vi "RT Loop - Pumps.vi"(11 "Message Queue":refnum<queue>) -> ()   [LabVIEW 2018]
doc: "This Control Loop VI performs control calculations of diverter line (DL) rotation."
uses:
  Support/Message Queue/Message Cluster.ctl
  Support/Message Queue/Message.ctl
  <vilib>/Platform/TimedLoop/XDataNode/timing_clust.ctl
  <vilib>/Platform/TimedLoop/XDataNode/nitl_modes.ctl
  <vilib>/Platform/TimedLoop/XDataNode/wakeup.ctl
  Controls/Pumps State.ctl
  <vilib>/Platform/TimedLoop/XDataNode/loadnilvce.vi
  Globals/Global - RT Channels.vi
  <vilib>/Platform/TimedLoop/XDataNode/XDataNode.xnode
  <vilib>/Platform/TimedLoop/XDataNode/XDNodeRunTimeDep.lvlib
  support/Message Queue/Message Queue.lvlib
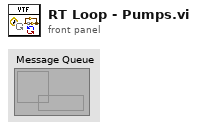
[diagram p1: front panel]
types:
  T1 = typedef "XDNodeRunTimeDep.lvlib/timing_clust.ctl" = cluster{"Expected End [f-1]":u64, "Actual End [f-1]":u64, "Finished Late? [f-1]":bool, "Expected End [i-1]":u64, "Actual End [i-1]":u64, "Finished Late? [i-1]":bool, "Expected Start [i]":u64, "Actual Start [i]":u64, "Expected Start [f]":u64, "Actual Start [f]":u64, "Source Name":string, "Structure Name":string, "Period":i64, "Deadline":i64, "Offset":i64, "Start":i64, "Priority":i32, "Timeout":i32, "Mode":T2, "Wakeup Reason":T3, "Error":errorcluster, "Source Type":string, "Secondary Source Type":string, "Global End Time":u64, "Global Start Time":u64, "Frame Duration":u64, "Iteration Duration":u64, "Assigned CPU":i32, "I/O Scan Engine Mode":u32}
  T2 = typedef "XDNodeRunTimeDep.lvlib/nitl_modes.ctl" = enum32{"No Change", "Process missed periods, maintain original phase", "Discard missed periods, maintain original phase", "Process missed periods, ignore original phase", "Discard missed periods, ignore original phase"}
  T3 = typedef "XDNodeRunTimeDep.lvlib/wakeup.ctl" = enum32{"Normal", "Aborted", "Asynchronous wakeup", "Timing source error", "Timed loop error", "Timeout"}
  T4 = typedef "Pumps State.ctl" = enum16{"Do Nothing", "Run Pump 1", "Run Pump 2", "Run Pump 3", "Run Pump 4", "Run Pump 5", "Stop Pump 1", "Stop Pump 2", "Stop Pump 3", "Stop Pump 4", "Stop Pump 5"}
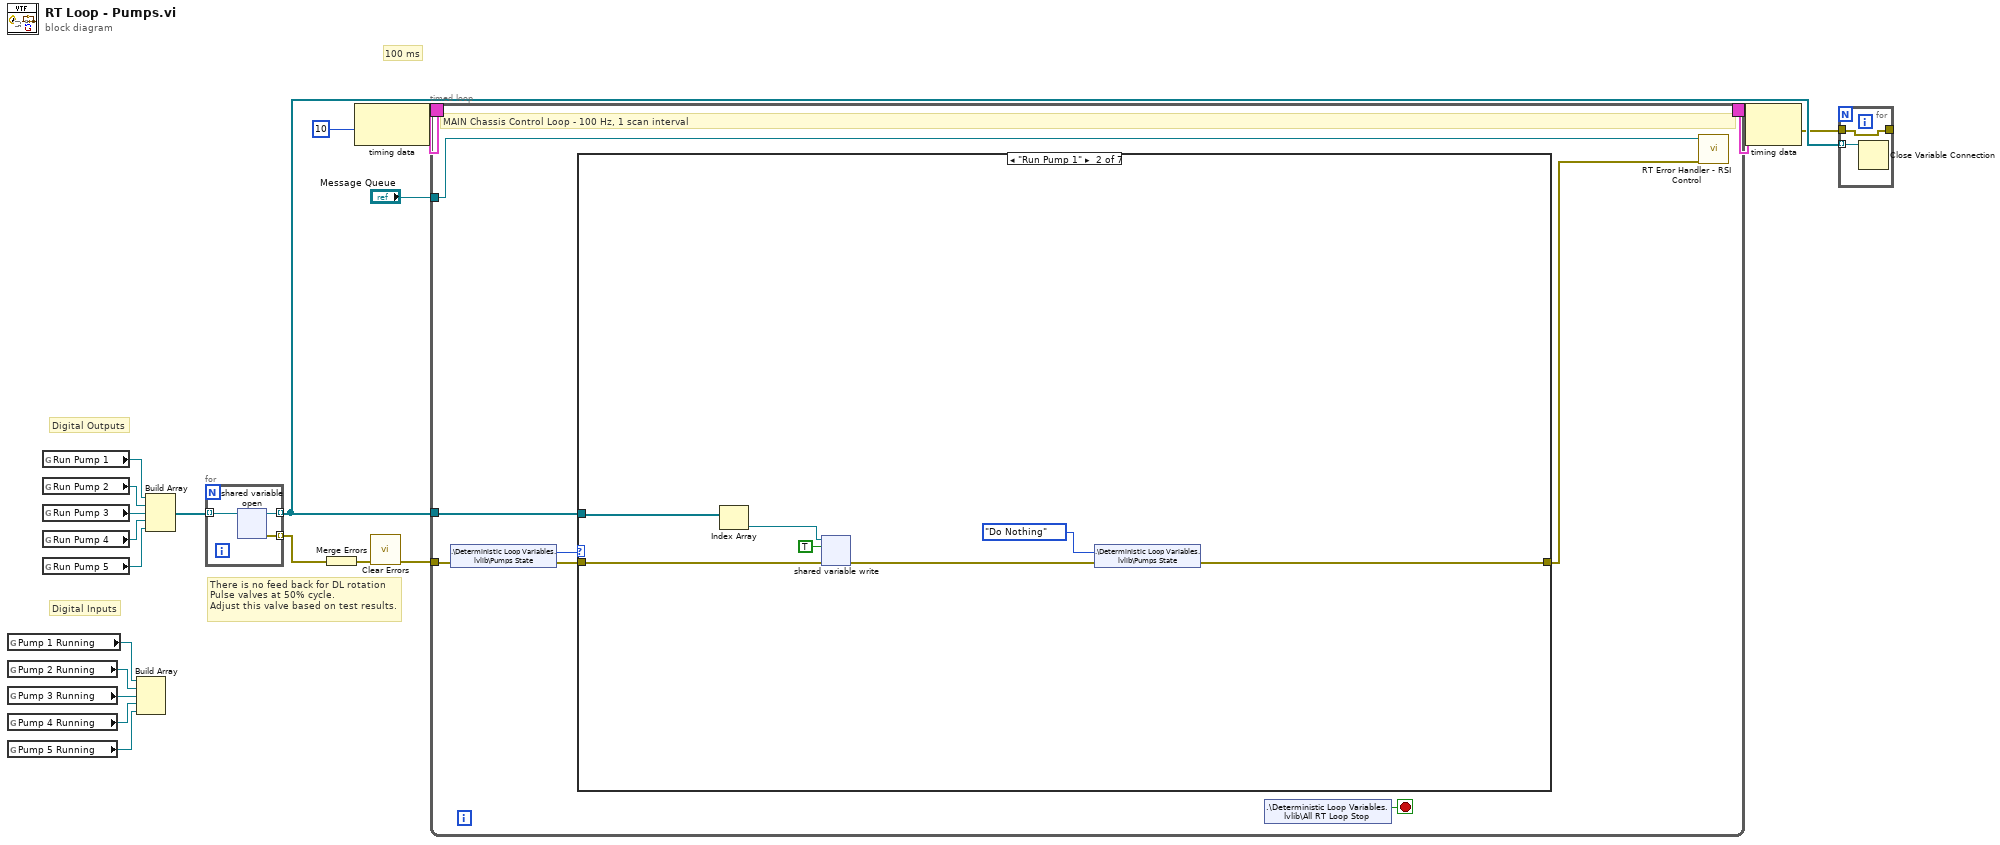
[diagram p0: block diagram]
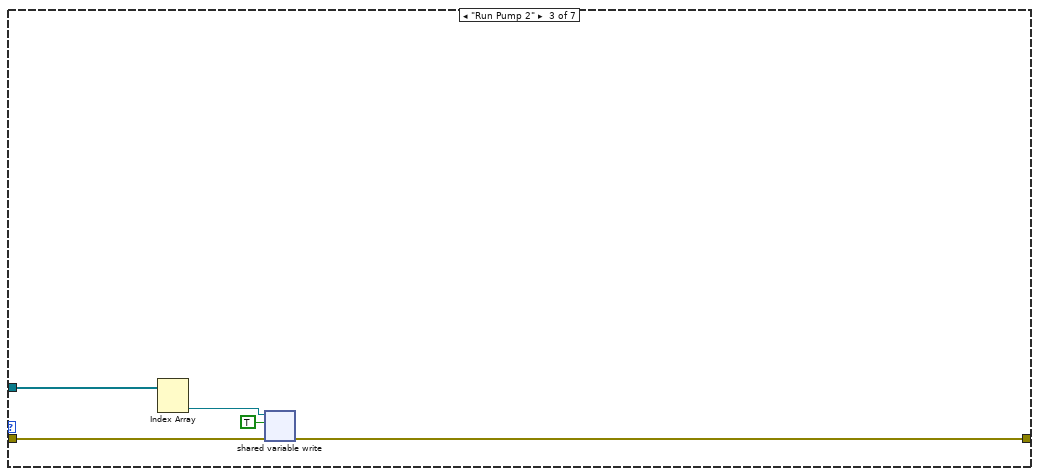
[diagram p3: hidden frame]
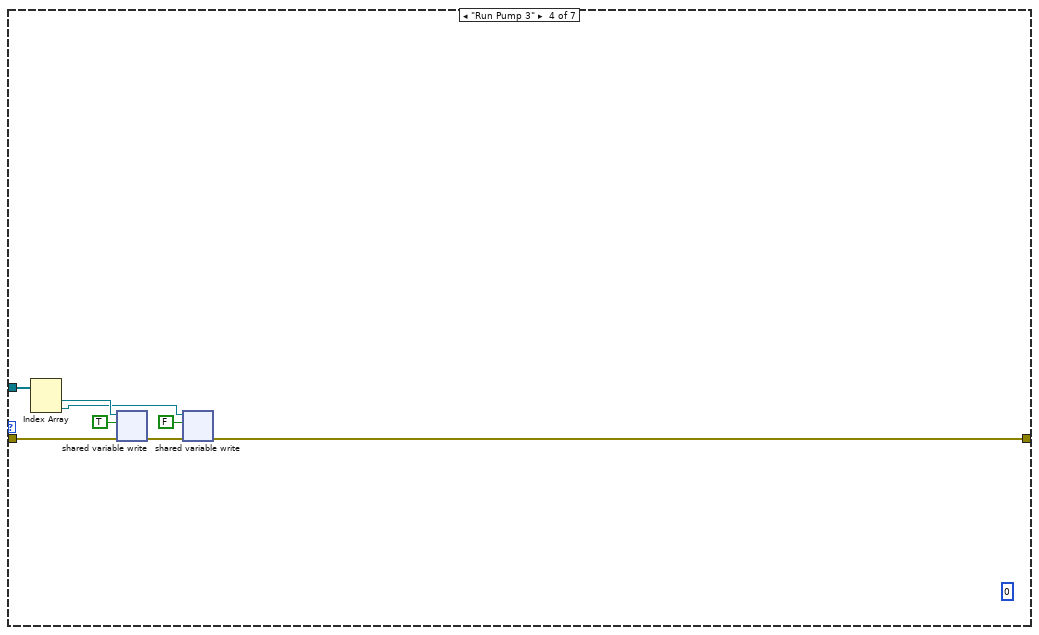
[diagram p4: hidden frame]
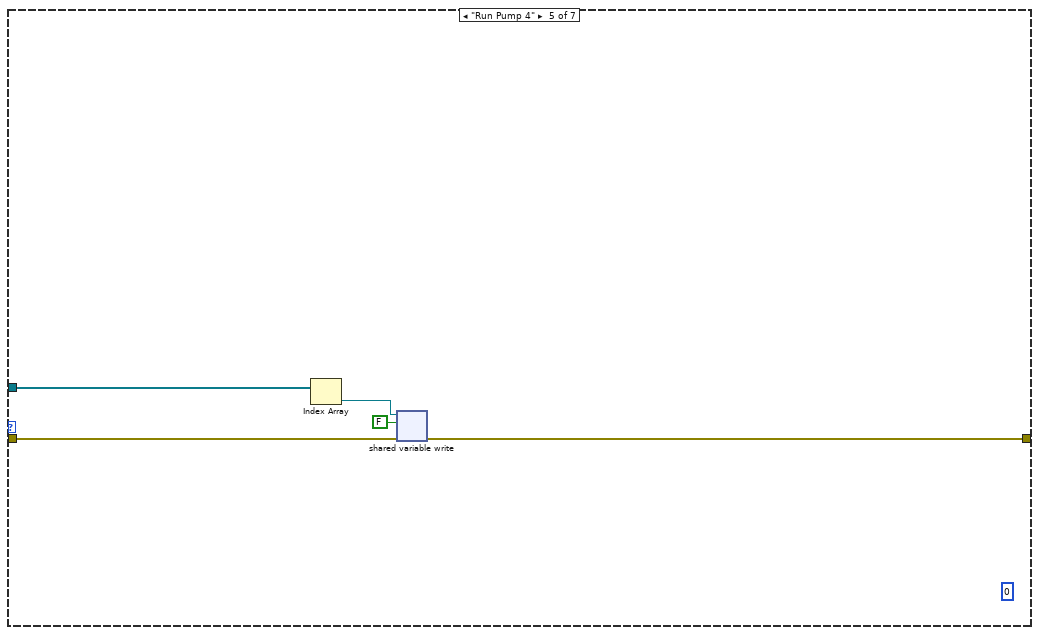
[diagram p5: hidden frame]
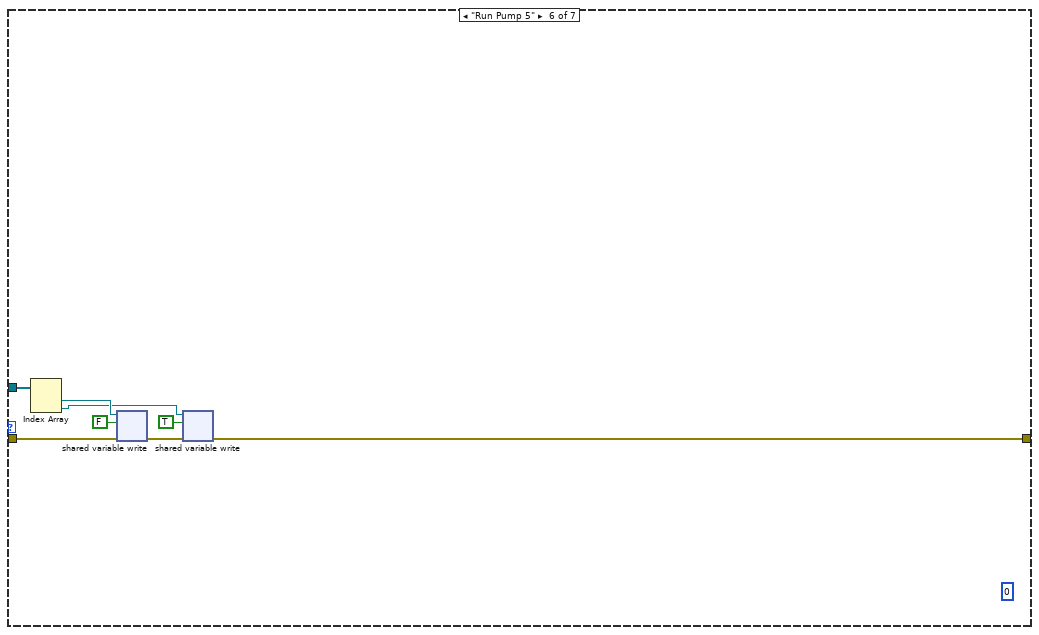
[diagram p6: hidden frame]
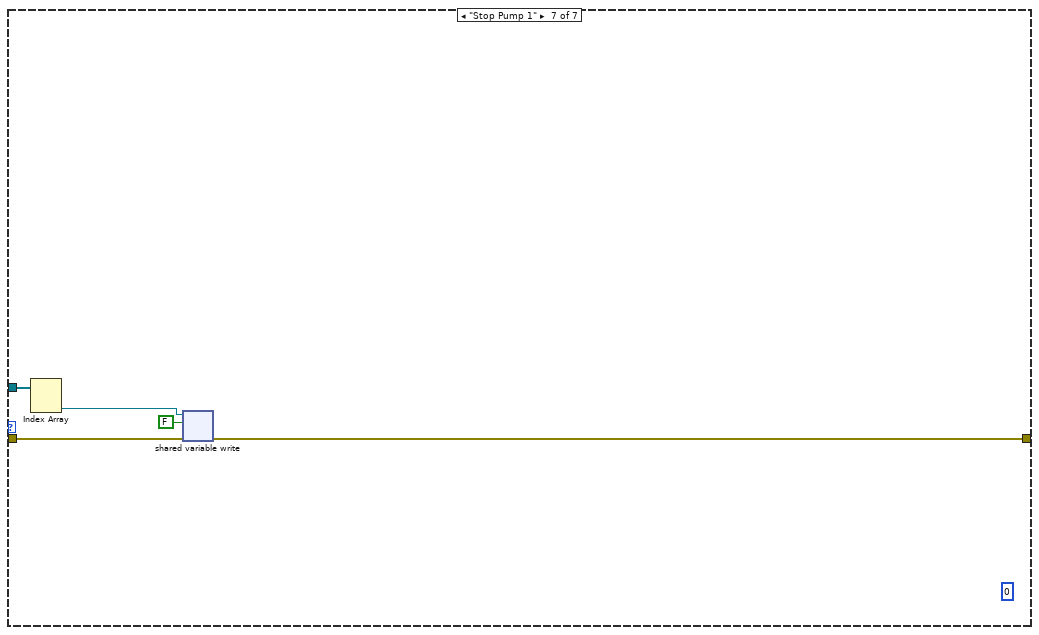
[diagram p7: hidden frame]
diagram:
  # "100 ms"
  # "Digital Inputs"
  # "There is no feed back for DL rotation\nPulse valves at 50% cycle. \nAdjust this valve based on test results."
  # "Digital Outputs"
  n1 = global read "Global - RT Channels.vi" "Pump 1 Running"() -> (w1:refnum<k21>)
  n2 = global read "Global - RT Channels.vi" "Pump 2 Running"() -> (w2:refnum<k21>)
  n3 = global read "Global - RT Channels.vi" "Pump 3 Running"() -> (w3:refnum<k21>)
  n4 = global read "Global - RT Channels.vi" "Pump 4 Running"() -> (w4:refnum<k21>)
  n5 = global read "Global - RT Channels.vi" "Pump 5 Running"() -> (w5:refnum<k21>)
  n6 = global read "Global - RT Channels.vi" "Run Pump 1"() -> (w11:refnum<k21>)
  n7 = global read "Global - RT Channels.vi" "Run Pump 2"() -> (w10:refnum<k21>)
  n8 = global read "Global - RT Channels.vi" "Run Pump 3"() -> (w9:refnum<k21>)
  n9 = global read "Global - RT Channels.vi" "Run Pump 4"() -> (w8:refnum<k21>)
  n10 = global read "Global - RT Channels.vi" "Run Pump 5"() -> (w7:refnum<k21>)
  n11 = Build Array(w1, w2, w3, w4, w5) -> ()  [unwired: 1 out]
  n12 = Build Array(w11, w10, w9, w8, w7) -> (w6:refnum<k21>[])
  n13 = for {
    tunnel: w6 -> [w23] mode=indexing
    tunnel: [w22] -> w15 mode=indexing
    tunnel: [w21] -> w12 mode=indexing
    n14 = shared-variable-open(w23) -> (w22:refnum<k21>, w21:errorcluster)  [unwired: 1 in]
  }
  n15 = Merge Errors(w12) -> (w13:errorcluster)
  n16 = node-c288(i64 10 ("Period")) -> (w20:T1)
  n17 = call <vilib>:"Clear Errors.vi"("error in (no error)"=w13) -> ("error out"=w16:errorcluster)  [unwired: 5 in, 1 out]
  n18 = timed-loop {
    timing: w20 -> [_]
    timing-out: [_] -> w19
    tunnel: "Message Queue" -> [w25]
    tunnel: w16 -> [w27]
    tunnel: w15 -> [w29]
    stop <- w30 stop-if-true
    # "MAIN Chassis Control Loop - 100 Hz, 1 scan interval"
    n19 = shared-variable ".\\Deterministic Loop Variables.lvlib\\Pumps State"(error in=w27) -> (w28:T4, error out=w26:errorcluster)
    n20 = case shown="\"Run Pump 1\"" w28 {
      tunnel: w29 -> [_ w38 w42 w51 w56 w64 w69]
      tunnel: w26 -> [w31 w36 w40 w48 w54 w61 w67]
      tunnel: [w31 w33 w43 w44 w53 w57 w66] -> w24
      frame "Do Nothing", Default {
      }
      frame "Run Pump 1" {
        n21 = Index Array(array=w38) -> (element=w37:refnum<k21>)  [unwired: 1 in]
        n22 = shared-variable-write(w37, w36, TRUE ("data in")) -> (w34:errorcluster)  [unwired: 1 out]
        n23 = shared-variable ".\\Deterministic Loop Variables.lvlib\\Pumps State"(Pumps_State."Do Nothing" ("Pumps State"), error in=w34) -> (error out=w33:errorcluster)
      }
      frame "Run Pump 2" {
        n24 = Index Array(array=w42) -> (element #2=w41:refnum<k21>)  [unwired: 2 in, 1 out]
        n25 = shared-variable-write(w41, w40, TRUE ("data in")) -> (w43:errorcluster)  [unwired: 1 out]
      }
      frame "Run Pump 3" {
        (unwired) 0
        n26 = Index Array(array=w51) -> (element #1=w50:refnum<k21>, element #2=w49:refnum<k21>)  [unwired: 2 in]
        n27 = shared-variable-write(w50, w48, TRUE ("data in")) -> (w47:errorcluster)  [unwired: 1 out]
        n28 = shared-variable-write(w49, w47, FALSE ("data in")) -> (w44:errorcluster)  [unwired: 1 out]
      }
      frame "Run Pump 4" {
        (unwired) 0
        n29 = Index Array(array=w56) -> (element=w55:refnum<k21>)  [unwired: 1 in]
        n30 = shared-variable-write(w55, w54, FALSE ("data in")) -> (w53:errorcluster)  [unwired: 1 out]
      }
      frame "Run Pump 5" {
        (unwired) 0
        n31 = Index Array(array=w64) -> (element #1=w63:refnum<k21>, element #2=w62:refnum<k21>)  [unwired: 2 in]
        n32 = shared-variable-write(w63, w61, FALSE ("data in")) -> (w60:errorcluster)  [unwired: 1 out]
        n33 = shared-variable-write(w62, w60, TRUE ("data in")) -> (w57:errorcluster)  [unwired: 1 out]
      }
      frame "Stop Pump 1" {
        (unwired) 0
        n34 = Index Array(array=w69) -> (element #2=w68:refnum<k21>)  [unwired: 2 in, 1 out]
        n35 = shared-variable-write(w68, w67, FALSE ("data in")) -> (w66:errorcluster)  [unwired: 1 out]
      }
    }
    n36 = shared-variable ".\\Deterministic Loop Variables.lvlib\\All RT Loop Stop"() -> (w30:bool)  [unwired: 1 in, 1 out]
    n37 = call "RT Error Handler - RSI Control.vi"("error in (no error)"=w24, "Message Queue"=w25) -> ()  [unwired: 8 in, 2 out]
  }
  n38 = node-c288(w19) -> (w14:errorcluster)
  n39 = for {
    tunnel: w14 -> [w72]
    tunnel: w15 -> [w73] mode=indexing
    tunnel: [w72] -> _
    n40 = Close Variable Connection(11:w73) -> ()  [unwired: 1 in, 1 out]
  }
